vi "Close.vi"(8 "error in (no error)":errorcluster, 11 "WebSocket Client in":refnum<class "WebSocket Client.lvclass">) -> (0 "error out":errorcluster, 3 "WebSocket Client out":refnum<class "WebSocket Client.lvclass">)   [LabVIEW 2021, in "WebSockets.lvlib" / "WebSocket Client.lvclass"]
doc: "Opens a conenction and creates a new WebSocket Client using the NI VISA TCP Socket.\nWebSockets 2.0.1.40\nSam Sharp - MediaMongrels Ltd\nCopyright (c) 2019, MediaMongrels Ltd"
uses:
  WebSocket Client.lvclass
  WebSocket Client.lvclass/WebSocket Client.ctl
  WebSocket/WebSocket.lvclass
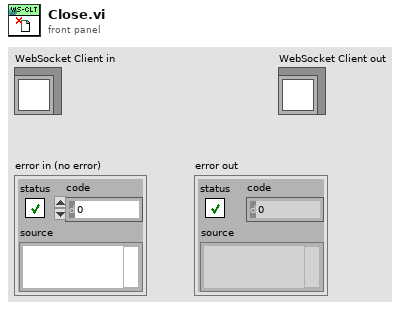
[diagram p1: front panel]
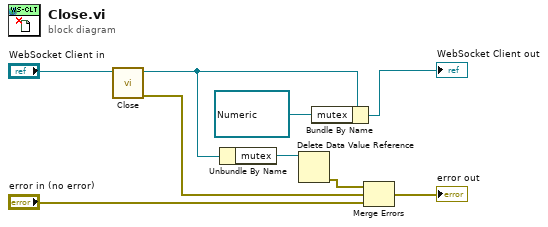
[diagram p0: block diagram]
diagram:
  n1 = call-parent "Close.vi"("WebSocket in"="WebSocket Client in") -> ("error out"=w4:errorcluster, "WebSocket out"=w3:refnum<class "WebSocket Client.lvclass">)  [unwired: 9 in]
  n2 = Unbundle By Name(w3) -> ("mutex"=w9:refnum<data-value>)
  n3 = Delete Data Value Reference(data value reference=w9) -> (error out=w8:errorcluster)  [unwired: 1 in, 1 out]
  n4 = Bundle By Name(cluster=w3, "mutex"=refnum<data-value> refnum) -> (→"WebSocket Client out":refnum<class "WebSocket Client.lvclass">)
  n5 = Merge Errors(w8, w4, "error in (no error)") -> (→"error out":errorcluster)
